vi "Database - Add Entry.vi"(0 "reference in":refnum<class "Database_UUT.lvclass">, 9 "Part Number":string, 11 "error in (no error)":errorcluster, 12 "Property Labels":string[](array[string]), 13 "Property Values":string[](array[string]), 14 "Datatype":T1[](array[typedef])) -> (4 "reference out":refnum<class "Database_UUT.lvclass">, 15 "error out":errorcluster)   [LabVIEW 2017, in "Database_UUT.lvclass"]
uses:
  Database_UUT.lvclass
  TypeDefs/Datatype.ctl
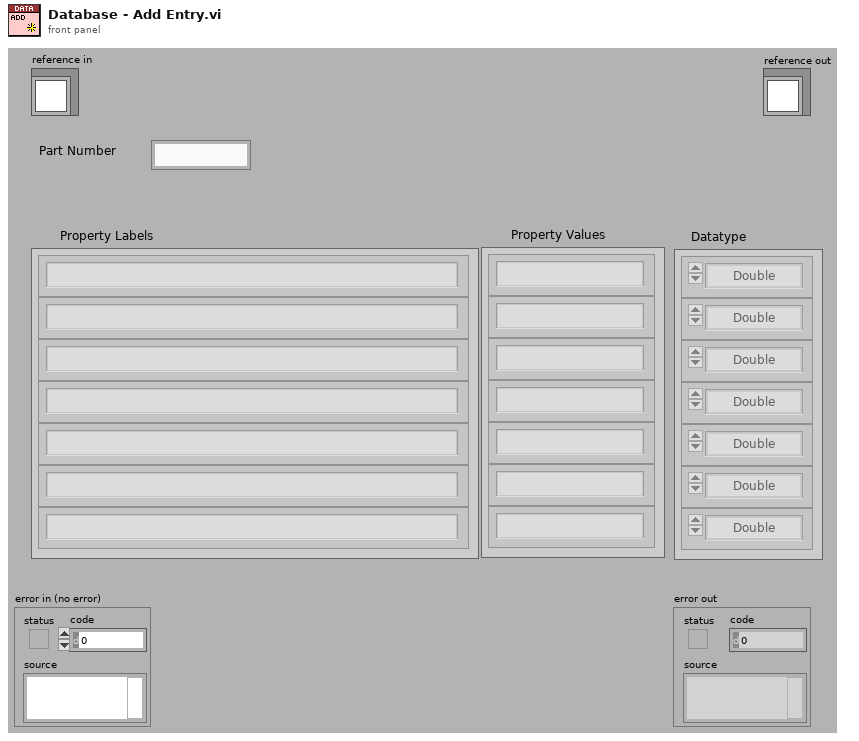
[diagram p1: front panel]
types:
  T1 = typedef "Database_UUT.lvclass/Datatype.ctl" = enum16{"Double", "Int32", "Text String", "Bool (0 or 1)"}
  T2 = enum16{"open", "open or create", "create or replace", "create", "open (read-only)"}
  T3 = typedef "Database_UUT.lvclass/ObjectAttributes.ctl" = cluster{"Filepath to Database":path}
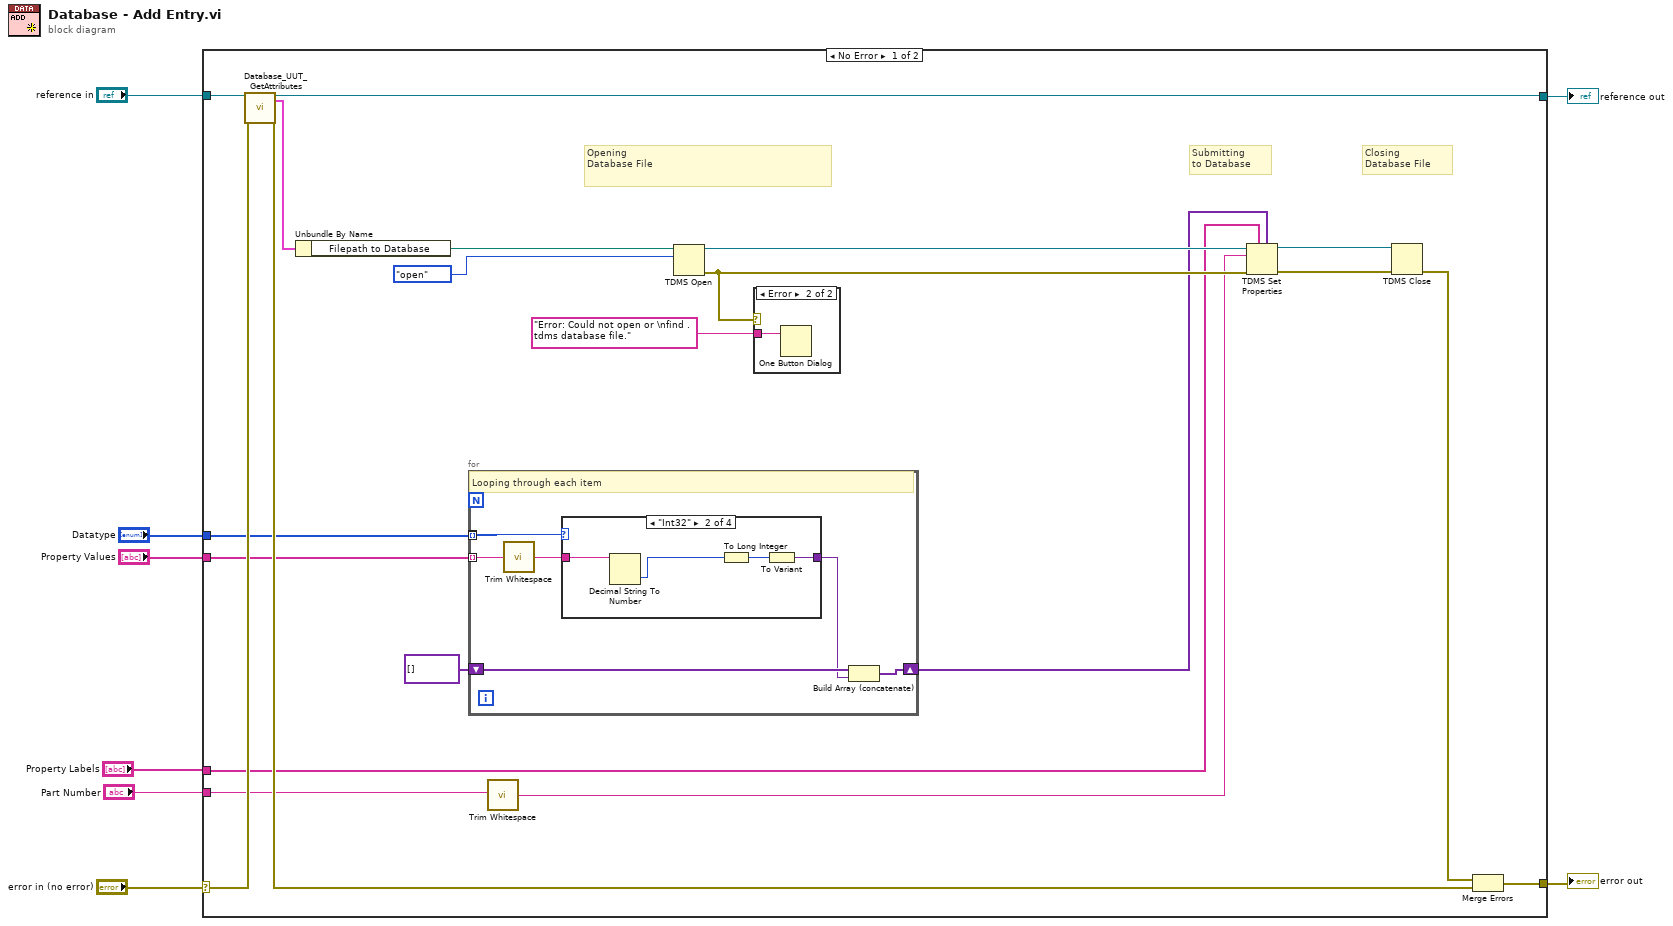
[diagram p0: block diagram]
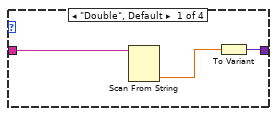
[diagram p2: hidden frame]
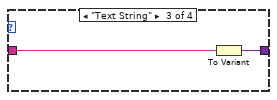
[diagram p3: hidden frame]
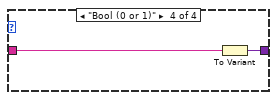
[diagram p4: hidden frame]
diagram:
  n1 = case shown="No Error" "error in (no error)" {
    selector: "error in (no error)" -> [w28 w49]
    tunnel: [w20 w49] -> w7
    tunnel: [w26 w48] -> w5
    tunnel: "reference in" -> [w29 w48]
    tunnel: "Part Number" -> [w10 _]
    tunnel: "Property Labels" -> [w15 _]
    tunnel: "Property Values" -> [w14 _]
    tunnel: "Datatype" -> [w12 _]
    frame No Error {
      # "Submitting\nto Database"
      # "Closing \nDatabase File"
      # "Opening\nDatabase File"
      n2 = call "Database_UUT_GetAttributes.vi"("reference in"=w29, "error in (no error)"=w28) -> ("reference out"=w26:refnum<class "Database_UUT.lvclass">, "Data"=w27:T3, "error out"=w19:errorcluster)  [unwired: 14 in, 1 out]
      n3 = Unbundle By Name(w27) -> ("Filepath to Database"=w24:path)
      n4 = for {
        tunnel: w14 -> [w31] mode=indexing
        shift-right: [w35] -> w13
        shift-left: variant[] [] -> [w34]
        tunnel: [w33] -> _ mode=indexing
        tunnel: w12 -> [w33] mode=indexing
        # "Looping through each item"
        n5 = call <vilib>:"Trim Whitespace.vi"("string"=w31) -> ("trimmed string"=w30:string)  [unwired: 1 in]
        n6 = case shown="\"Int32\"" w33 {
          tunnel: w30 -> [w37 w41 w43 w45]
          tunnel: [w38 w42 w44 w46] -> w32
          frame "Double", Default {
            n7 = Scan From String(input string=w37) -> (output 1=w36:dbl)  [unwired: 4 in, 3 out]
            n8 = To Variant(anything=w36) -> (Variant=w38:variant)
          }
          frame "Int32" {
            n9 = Decimal String To Number(string=w41) -> (number=w40:i32)  [unwired: 2 in, 1 out]
            n10 = To Long Integer(number=w40) -> (32bit integer=w39:i32)
            n11 = To Variant(anything=w39) -> (Variant=w42:variant)
          }
          frame "Text String" {
            n12 = To Variant(anything=w43) -> (Variant=w44:variant)
          }
          frame "Bool (0 or 1)" {
            n13 = To Variant(anything=w45) -> (Variant=w46:variant)
          }
        }
        n14 = Build Array (concatenate)(w34, w32) -> (w35:variant[])
      }
      n15 = call <vilib>:"Trim Whitespace.vi"("string"=w10) -> ("trimmed string"=w9:string)  [unwired: 1 in]
      n16 = TDMS Open(10:T2."open" ("operation (0:open)"), 11:w24) -> (0:w16:errorcluster, 3:w23:refnum<k34>)  [unwired: 5 in]
      n17 = case shown="Error" w16 {
        tunnel: "Error: Could not open or \nfind .tdms database file." -> [_ w47]
        frame No Error {
        }
        frame Error {
          n18 = One Button Dialog(message=w47) -> ()  [unwired: 1 in, 1 out]
        }
      }
      n19 = TDMS Set Properties(5:w13, 7:w15, 8:w16, 10:w9, 11:w23) -> (0:w21:errorcluster, 3:w22:refnum<k34>)  [unwired: 1 in, 2 out]
      n20 = TDMS Close(8:w21, 11:w22) -> (0:w18:errorcluster)  [unwired: 1 out]
      n21 = Merge Errors(w18, w19) -> (w20:errorcluster)
    }
    frame Error {
    }
  }
  "error out" <- w7
  "reference out" <- w5
